vi "setData.vi"(8 "error in (no error)":errorcluster, 10 "Theme":T1, 11 "Theme in":refnum<class "Theme.lvclass">) -> (0 "error out":errorcluster, 3 "Theme out":refnum<class "Theme.lvclass">)   [LabVIEW 2017, in "Theme.lvlib" / "Theme.lvclass"]
uses:
  Theme.lvclass
  Private Data.ctl
  Theme.Colors/Theme.Colors.lvclass
  Theme.Font/Theme.Font.lvclass
  Theme.lvclass/Theme.ctl
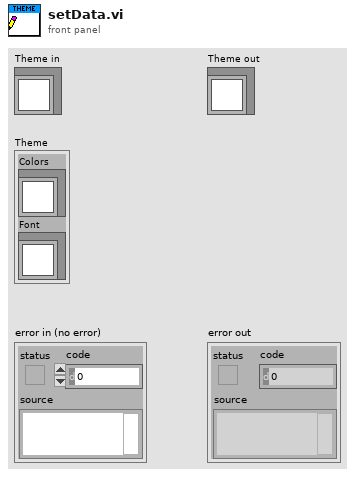
[diagram p1: front panel]
types:
  T1 = typedef "Theme.lvlib/Theme.lvclass/Private Data.ctl" = cluster{"Colors":refnum<class "Theme.Colors.lvclass">, "Font":refnum<class "Theme.Font.lvclass">}
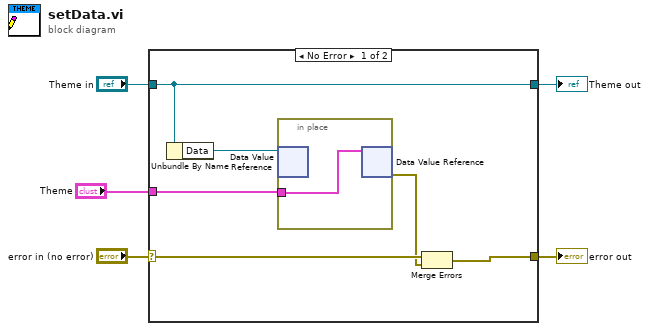
[diagram p0: block diagram]
diagram:
  n1 = case shown="No Error" "error in (no error)" {
    selector: "error in (no error)" -> [w11 w13]
    tunnel: [w8 w13] -> w3
    tunnel: [w10 w14] -> w4
    tunnel: "Theme in" -> [w10 w14]
    tunnel: "Theme" -> [w6 _]
    frame No Error {
      n2 = Unbundle By Name(w10) -> ("Data"=w9:refnum<data-value>)
      n3 = in-place {
        in-place-border: w6 -> [w12]
        n4 = in-place-dvr #1(w9) -> ()  [unwired: 2 out]
        n5 = in-place-dvr #1(w12) -> (w7:errorcluster)  [unwired: 1 out]
      }
      n6 = Merge Errors(w11, w7) -> (w8:errorcluster)
    }
    frame Error {
    }
  }
  "error out" <- w3
  "Theme out" <- w4
